vi "testInsertIndexOne.vi"(8 "error in (no error)":errorcluster, 11 "TestCase in":refnum<class "ListImp_Empty.lvclass">) -> (0 "error out":errorcluster, 3 "TestCase out":refnum<class "ListImp_Empty.lvclass">)   [LabVIEW 2013, in "ListImp_Empty.lvclass"]
uses:
  ListImp_Empty.lvclass
  ListImp_Empty.lvclass/ListImp_Empty.ctl
  source/LapDog.Collections.Lists/ListImp/ListImp.lvclass
  <vilib>/addons/_JKI Toolkits/VI Tester/TestCase.llb/TestCase.lvclass
  UnitTestComparisons/UnitTestComparisons.lvlib
  source/LapDog.Collections.Common/I32/I32.lvclass
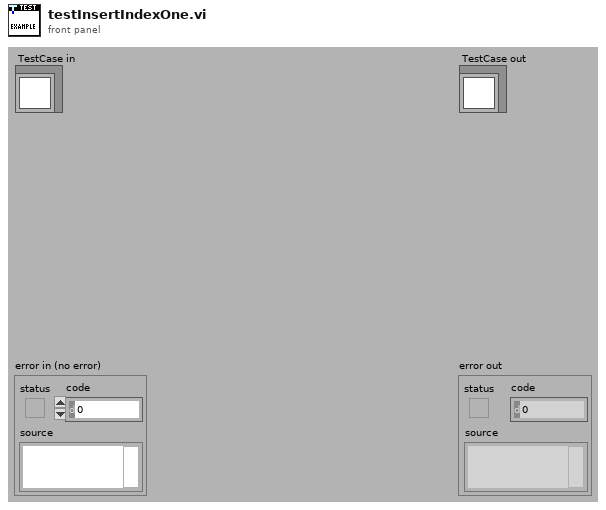
[diagram p1: front panel]
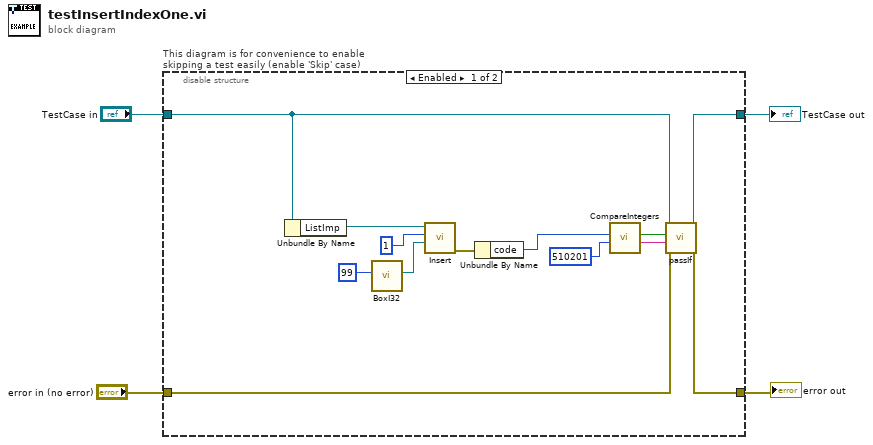
[diagram p0: block diagram]
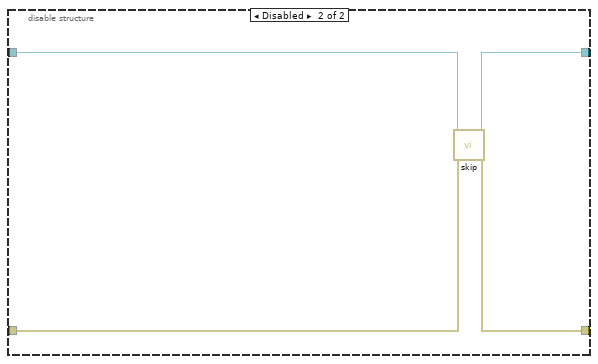
[diagram p2: hidden frame]
diagram:
  n1 = disable-structure "This diagram is for convenience to enable skipping a test easily (enable 'Skip' case)" shown="Enabled" {
    disable-tunnel: "TestCase in" -> [w14 w21]
    disable-tunnel: [w17 w19] -> w1
    disable-tunnel: [w16 w20] -> w3
    disable-tunnel: "error in (no error)" -> [w15 w18]
    frame Enabled {
      n2 = Unbundle By Name(w14) -> ("ListImp"=w8:refnum<class "ListImp.lvclass">)
      n3 = call "BoxI32.vi"("Numeric"=99) -> ("I32 out"=w5:refnum<class "I32.lvclass">)  [unwired: 10 in]
      n4 = call-dynamic "Insert.vi"("Item"=w5, "Index"=1, "ListImp in"=w8) -> ("error out"=w10:errorcluster)  [unwired: 7 in, 1 out]
      n5 = Unbundle By Name(w10) -> ("code"=w9:i32)
      n6 = call "CompareIntegers.vi"("Expected Value"=510201, "Actual Value"=w9) -> ("Message"=w12:string, "Equal?"=w13:bool)  [unwired: 8 in]
      n7 = call-dynamic "passIf.vi"("error in (no error)"=w15, "message (\"\")"=w12, "pass"=w13, "TestCase in"=w14) -> ("error out"=w16:errorcluster, "TestCase out"=w17:refnum<class "ListImp_Empty.lvclass">)  [unwired: 6 in]
    }
    frame Disabled {
      # "skip test result while test is under development"
      n8 = call <vilib>:"skip.vi"("error in (no error)"=w18, "TestCase in"=w21) -> ("error out"=w20:errorcluster, "TestCase out"=w19:refnum<class "ListImp_Empty.lvclass">)  [unwired: 8 in]
    }
  }
  "error out" <- w3
  "TestCase out" <- w1
